vi "Compute.vi"(8 "error in (no error)":errorcluster, 9 "Data Channels":T3, 10 "x-var":T2(array[cluster]), 11 "Multi in":refnum<class "Multi.lvclass">) -> (0 "error out":errorcluster, 1 "Add'l Data Channels":T3, 3 "Multi out":refnum<class "Multi.lvclass">)   [LabVIEW 2017, in "Multi.lvclass"]
doc: "Given a data channel and an x-coordinate, compute and return one or more new data channels."
uses:
  Multi.lvclass
  Instruments/Utility Classes/Readable/Data Channels.ctl
  Instruments/Utility Classes/Readable/Data Channel.ctl
  Instruments/Utility Classes/Readable/Data Point.ctl
  Instruments/Utility Classes/Readable/Time.ctl
  Instruments/Utility Classes/Readable/X.ctl
  Multi.lvclass/Multi.ctl
  Aux Data Source/Aux Data Source.lvclass
  Instruments/Utility Classes/Readable/Readable.lvclass
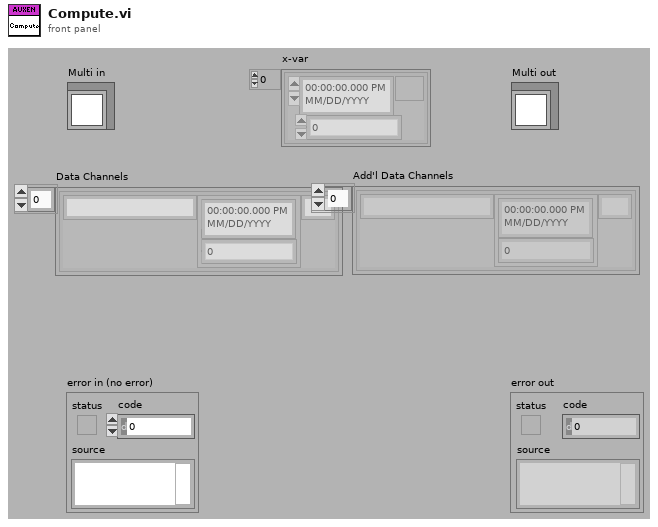
[diagram p1: front panel]
types:
  T1 = typedef "Readable.lvclass/X.ctl" = dbl
  T2 = cluster{"seconds since 1Jan1904":timestamp, "X-Var":T1}[]
  T3 = typedef "Readable.lvclass/Data Channels.ctl" = T4[]
  T4 = typedef "Readable.lvclass/Data Channel.ctl" = cluster{"Name":string, "Data Point":T5, "Unit":string}
  T5 = typedef "Readable.lvclass/Data Point.ctl" = cluster{"t":T6, "x":T1}
  T6 = typedef "Readable.lvclass/Time.ctl" = timestamp
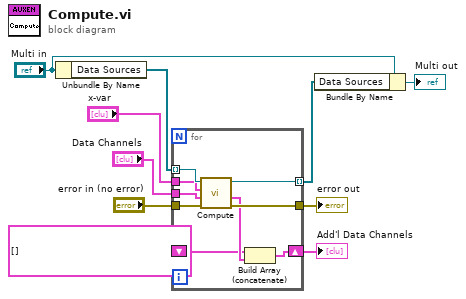
[diagram p0: block diagram]
diagram:
  n1 = Unbundle By Name("Multi in") -> ("Data Sources"=w10:refnum<class "Aux Data Source.lvclass">[])
  n2 = for {
    tunnel: w10 -> [w19] mode=indexing
    tunnel: [w18] -> w9 mode=indexing
    tunnel: "error in (no error)" -> [w17]
    tunnel: [w16] -> w5
    tunnel: "Data Channels" -> [w15]
    tunnel: "x-var" -> [w14]
    shift-right: [w13] -> w4
    shift-left: T3 [] ("Add'l Data Channels") -> [w11]
    n3 = call-dynamic "Compute.vi"("error in (no error)"=w17, "Data Channels"=w15, "x-var"=w14, "Aux Data Source in"=w19) -> ("error out"=w16:errorcluster, "Add'l Data Channels"=w12:T3, "Aux Data Source out"=w18:refnum<class "Aux Data Source.lvclass">)  [unwired: 5 in]
    n4 = Build Array (concatenate)(w11, w12) -> (w13:T3)
  }
  "error out" <- w5
  "Add'l Data Channels" <- w4
  n5 = Bundle By Name(cluster="Multi in", "Data Sources"=w9) -> (→"Multi out":refnum<class "Multi.lvclass">)
